vi "码原数组.vi"(1 "码元样本个数":i32=1000000, 2 "P(H0)":dbl=0.46) -> (0 "码元数组":dbl[](array[numeric]))   [LabVIEW 2020]
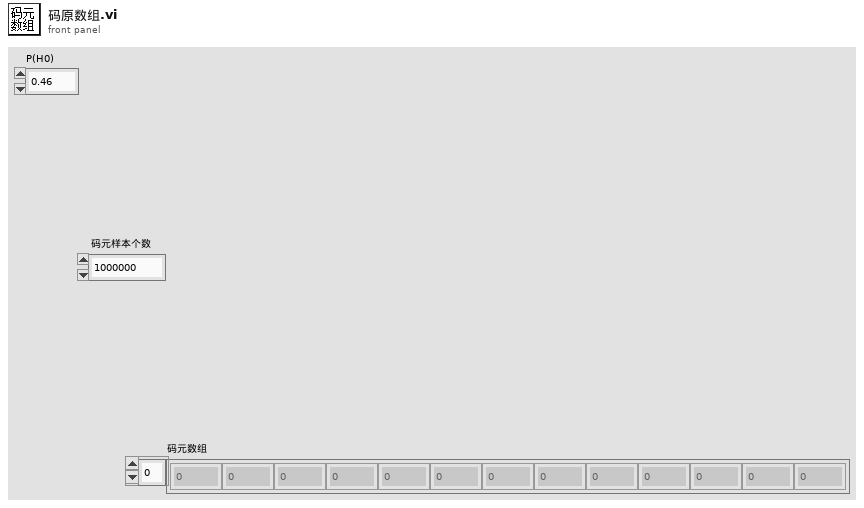
[diagram p1: front panel]
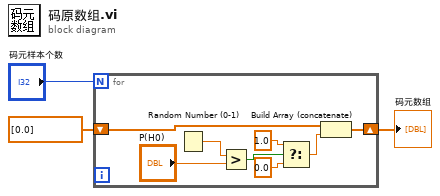
[diagram p0: block diagram]
diagram:
  n1 = for {
    N: "码元样本个数" -> [_]
    shift-right: [w7] -> w1
    shift-left: dbl[] [0.0] -> [w9]
    n2 = Random Number (0-1)() -> (number: 0 to 1=w6:dbl)
    n3 = Greater?(x=w6, y="P(H0)") -> (0:w11:bool)
    n4 = Select(t=1.0, s=w11, f=0.0) -> (s? t:f=w8:dbl)
    n5 = Build Array (concatenate)(w9, w8) -> (w7:dbl[])
  }
  "码元数组" <- w1
